vi "AutomatiskSMätare.vi"() -> ()   [LabVIEW 2020]
uses:
  <vilib>/Utility/file.llb/Write Delimited Spreadsheet (string).vi
panel:
  in  "SerialNumber alpha":string="27601609"
  in  "SerialNumber beta":string="27601582"
  in  "Offset gemensam":dbl=90.0
  in  "Offset beta":dbl=30.0
  in  "Offset alpha":dbl=-25.0
  out "betas":dbl[][](array[numeric])
  out "alphas":dbl[][](array[numeric])
  out "medelvärde":dbl[][](array[numeric])
  out "standardavvikelse":dbl[][](array[numeric])
  out "E-värden":dbl[](array[numeric])
  out "S-värde":dbl format="%.2f"
  in  "Antal mätningar":i32=6
  in  "Tidsfönster [s]":string="10"
  in  "Mitt av hysteres [V]":string="2.0"
  in  "Hysteresprocent [0|50|100]":string="100"
  in  "Trigger slope [POS|NEG]":string="POS"
  in  "GPIB Frekvensräknare":string="4"
  in  "Spara till fil":bool
  # "Inputs"
  # "Mätvärden"
  # "Vinklar"
  # "OBS! \nalla vinklar måste\nvara positiva"
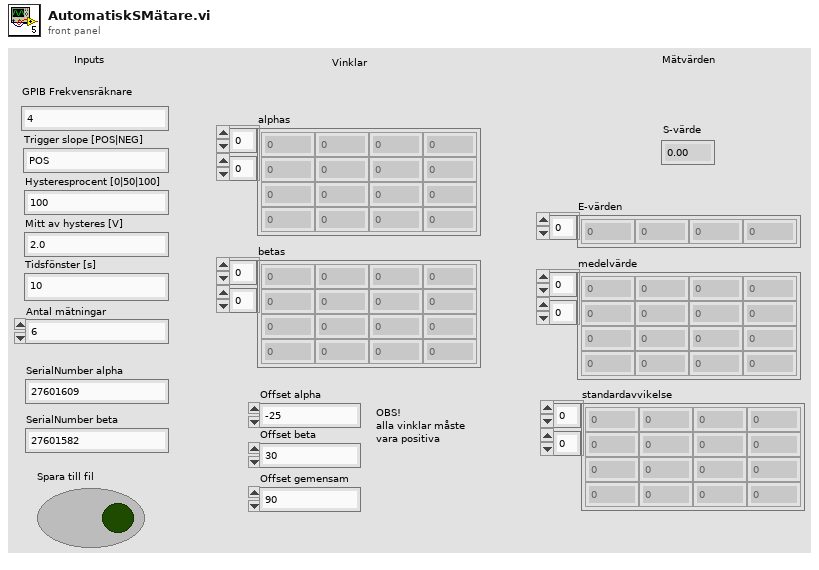
[diagram p1: front panel]
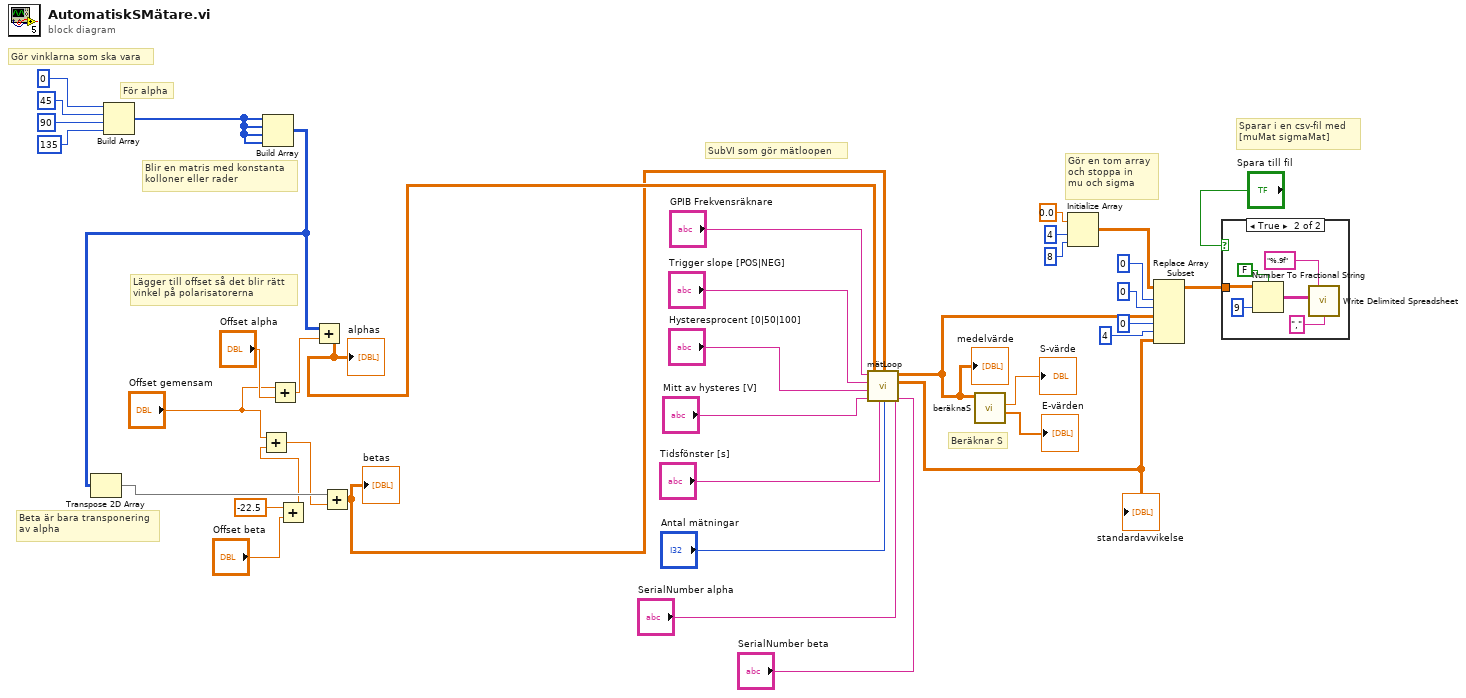
[diagram p0: block diagram]
diagram:
  # "Sparar i en csv-fil med \n[muMat sigmaMat]"
  # "Beräknar S"
  # "SubVI som gör mätloopen"
  # "Blir en matris med konstanta\nkolloner eller rader"
  # "Gör vinklarna som ska vara"
  # "Beta är bara transponering\nav alpha"
  # "Gör en tom array\noch stoppa in \nmu och sigma"
  # "För alpha"
  # "Lägger till offset så det blir rätt \nvinkel på polarisatorerna"
  n1 = Build Array(0, 45, 90, 135) -> (w24:i32[])
  n2 = Build Array(w24, w24, w24, w24) -> (w22:i32[][])
  n3 = Transpose 2D Array(2D array=w22) -> (transposed array=w23:i32[][])
  n4 = Add(x="Offset gemensam", y="Offset alpha") -> (x+y=w17:dbl)
  n5 = Add(x=-22.5, y="Offset beta") -> (x+y=w16:dbl)
  n6 = Add(x="Offset gemensam", y=w16) -> (x+y=w14:dbl)
  n7 = Add(x=w22, y=w17) -> (x+y=w20:dbl[][])
  "alphas" <- w20
  n8 = Add(x=w23, y=w14) -> (x+y=w19:dbl[][])
  "betas" <- w19
  n9 = call "mätLoop.vi"("SerialNumber beta"="SerialNumber beta", "SerialNumber alpha"="SerialNumber alpha", "Antal mätningar"="Antal mätningar", "beta"=w19, "Tidsfönster [s]"="Tidsfönster [s]", "alpha"=w20, "Mitt av hysteres [V]"="Mitt av hysteres [V]", "Hysteresprocent [0|50|100]"="Hysteresprocent [0|50|100]", "Trigger slope [POS|NEG]"="Trigger slope [POS|NEG]", "GPIB Frekvensräknare"="GPIB Frekvensräknare") -> ("standardavvikelse"=w1:dbl[][], "medelvärde"=w2:dbl[][])
  "standardavvikelse" <- w1
  "medelvärde" <- w2
  n10 = call "beräknaS.vi"("medelvärde"=w2) -> ("E-värden"=→"E-värden":dbl[], "S-värde"=→"S-värde":dbl)  [unwired: 9 in]
  n11 = Initialize Array(0.0 ("element"), 4 ("dimension size"), 8 ("dimension size")) -> (w6:dbl[][])
  n12 = Replace Array Subset(array=w6, new element #1=w2, index (row) #1=0 ("index (row)"), index (col) #1=0 ("disabled index (col)"), new element #2=w1, index (row) #2=0 ("index (row)"), index (col) #2=4 ("disabled index (col)")) -> (w3:dbl[][])
  n13 = case shown="True" "Spara till fil" {
    tunnel: w3 -> [_ w41]
    frame False {
    }
    frame True {
      n14 = Number To Fractional String(use system decimal point (T)=FALSE, number=w41, precision (6)=i16 9) -> (F-format string=w40:string[][])  [unwired: 1 in]
      n15 = call-poly <vilib>:"Write Delimited Spreadsheet.vi"("format (%s)"="%.9f" ("format (%.3f)"), "2D data"=w40, "delimiter (\\t)"="," ("delimiter (\\t)")) -> ()  [unwired: 11 in, 2 out]
    }
  }
